vi "myRIO_BRig_RT_dataMTrig_main__NoExp.vi"(0 "input_dataMTrig":u16[](array[numeric]), 2 "input_Audio_trig_L":bool, 3 "input_Audio_trig_R":bool, 4 "input_Laser_trig":bool, 5 "input_CueLed":bool) -> (14 "output_dataMTrig":u16[](array[numeric]), 16 "output_Audio_L":bool, 17 "output_Audio_R":bool, 18 "output_Laser":bool, 19 "output_CueLed":bool)   [LabVIEW 2014]
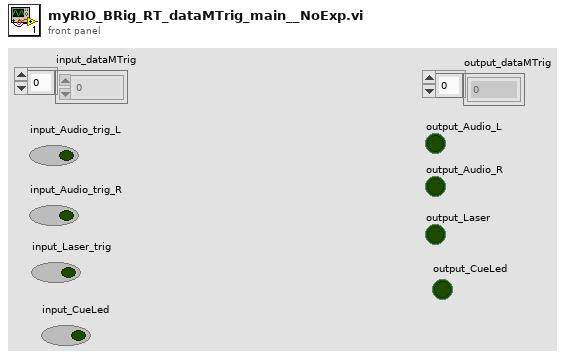
[diagram p1: front panel]
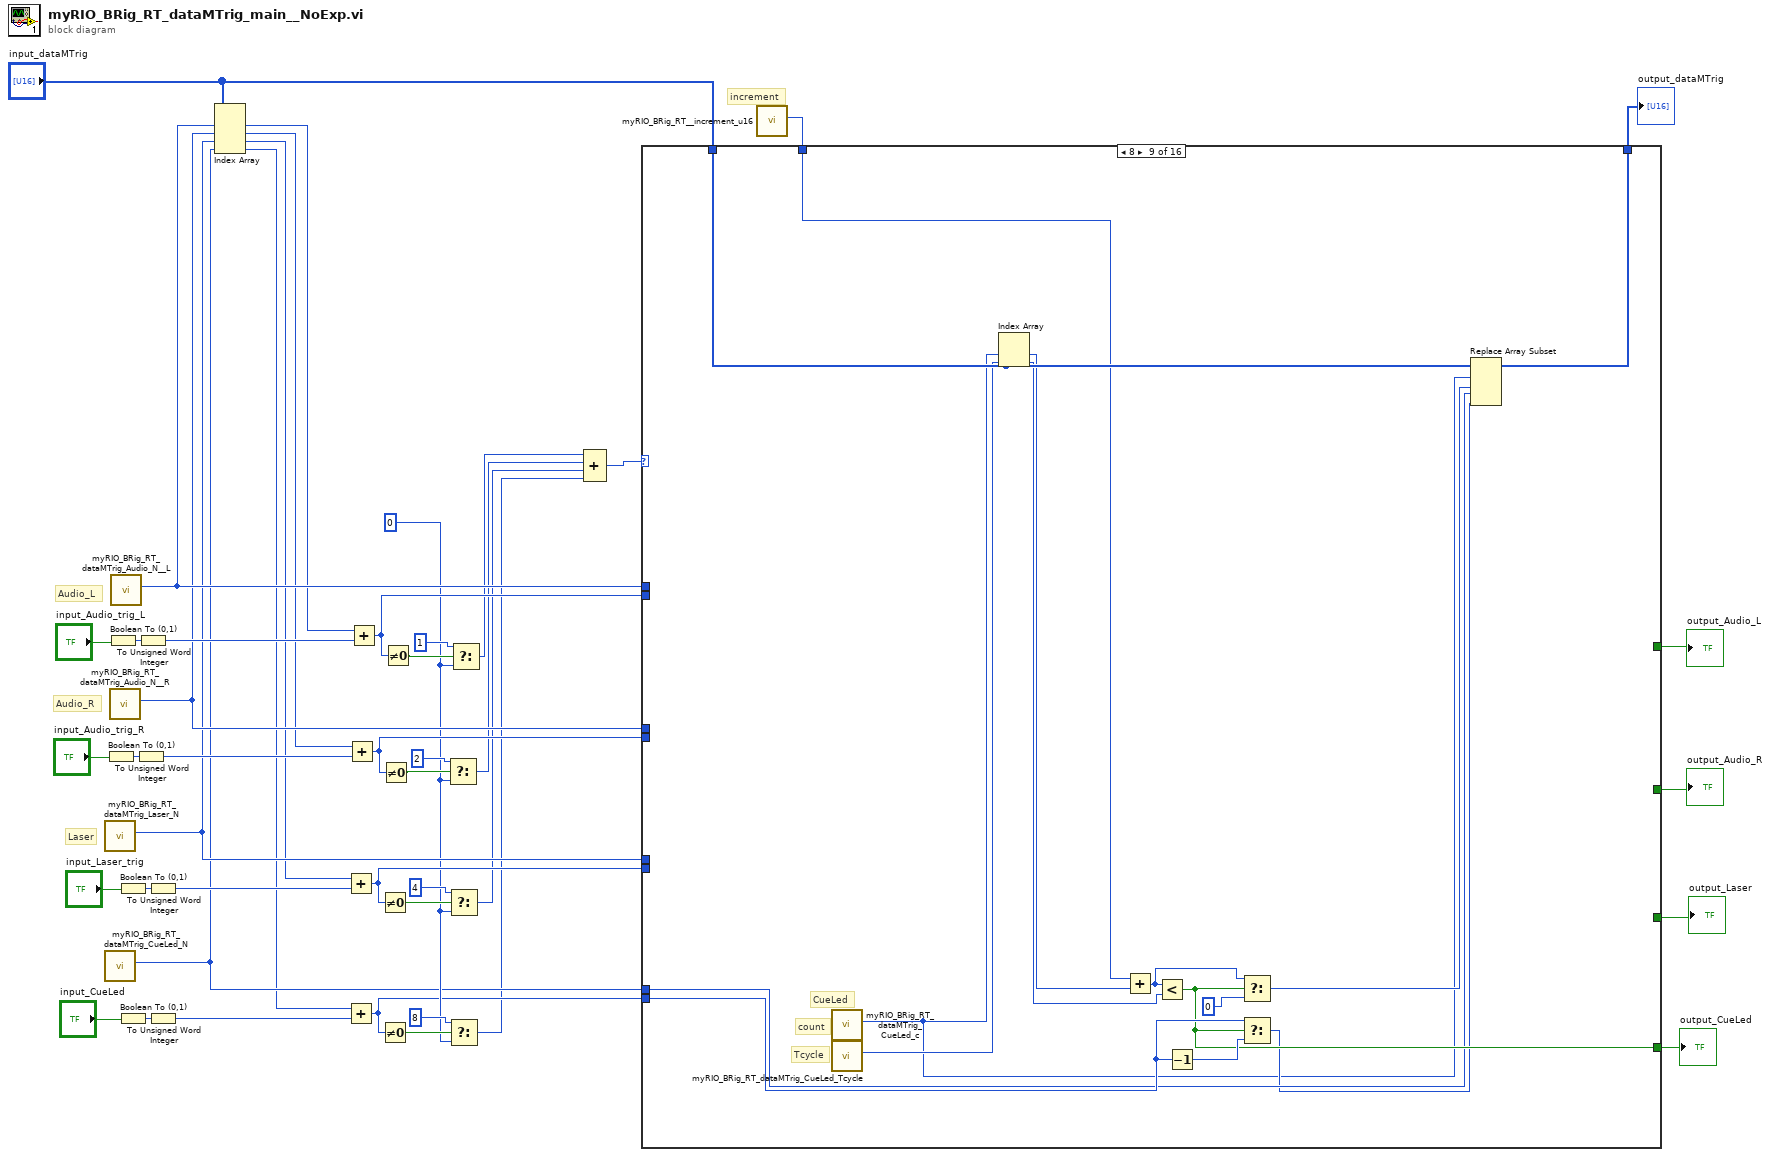
[diagram p0: block diagram]
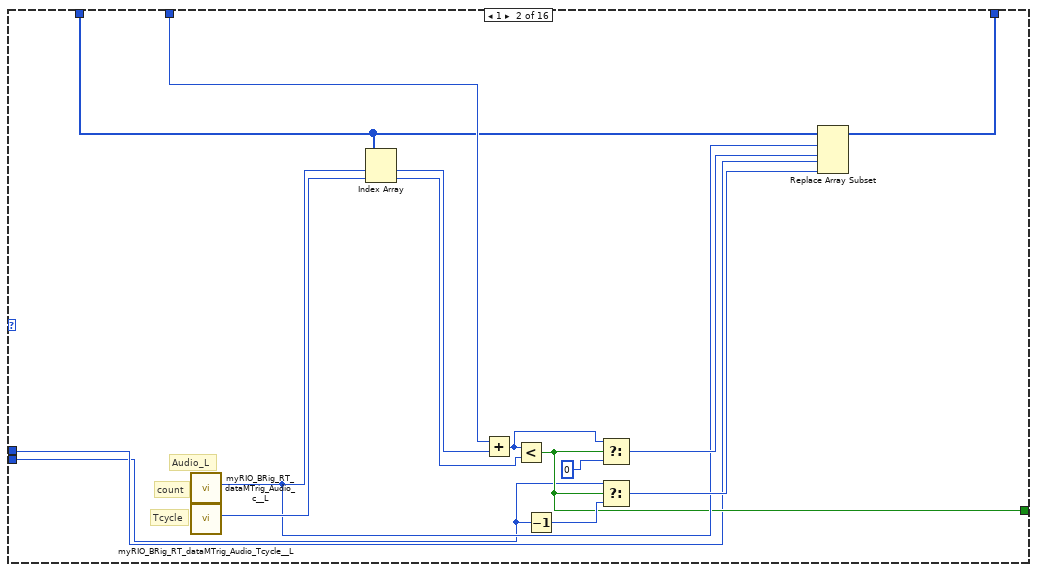
[diagram p3: hidden frame]
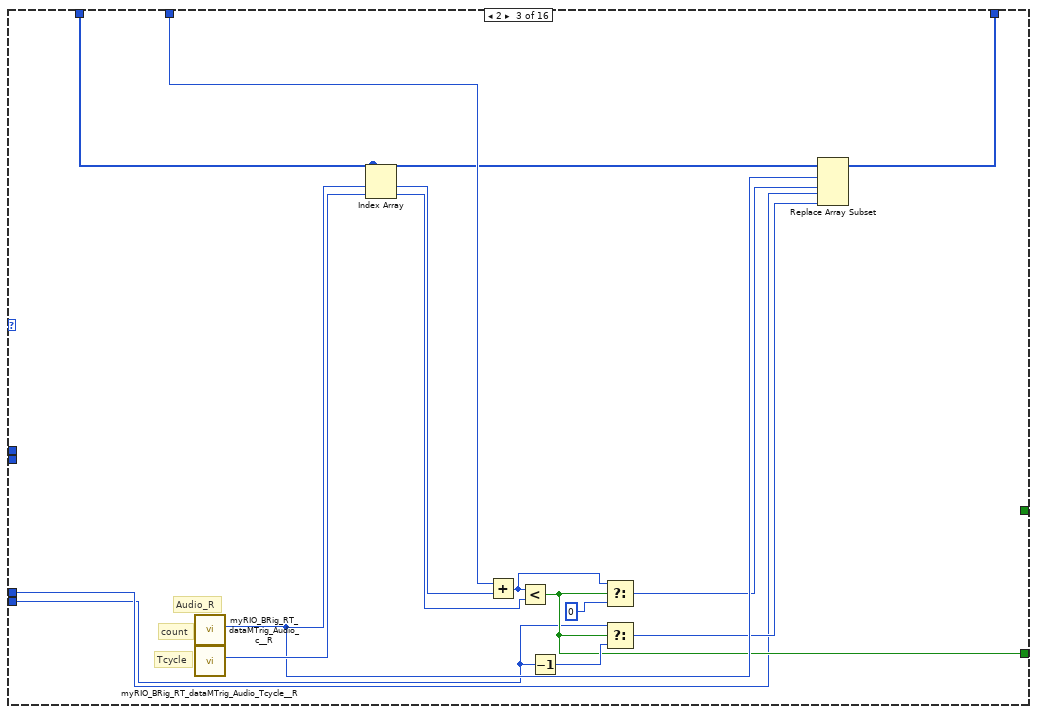
[diagram p4: hidden frame]
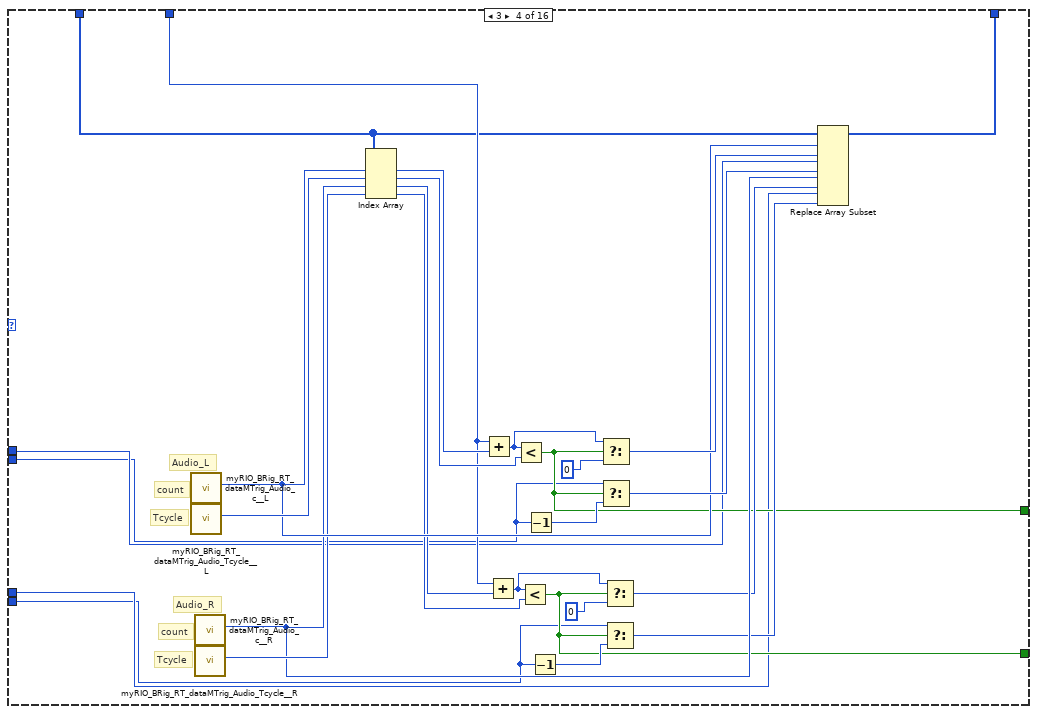
[diagram p5: hidden frame]
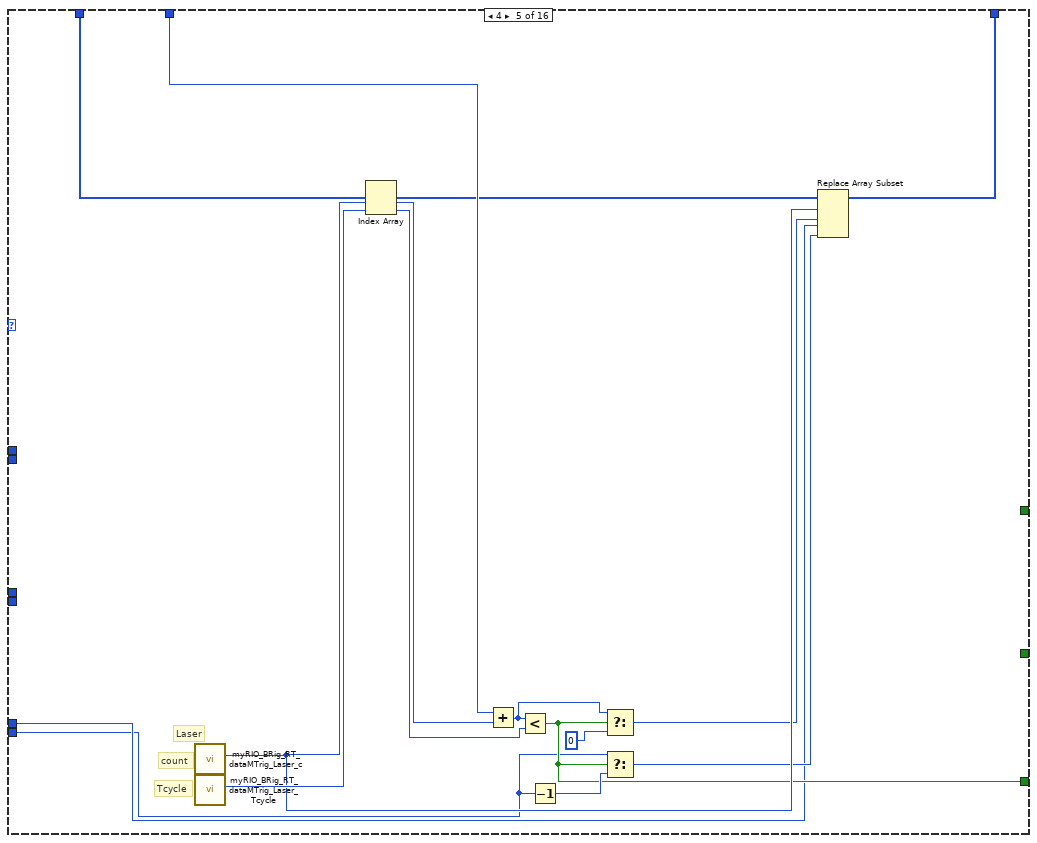
[diagram p6: hidden frame]
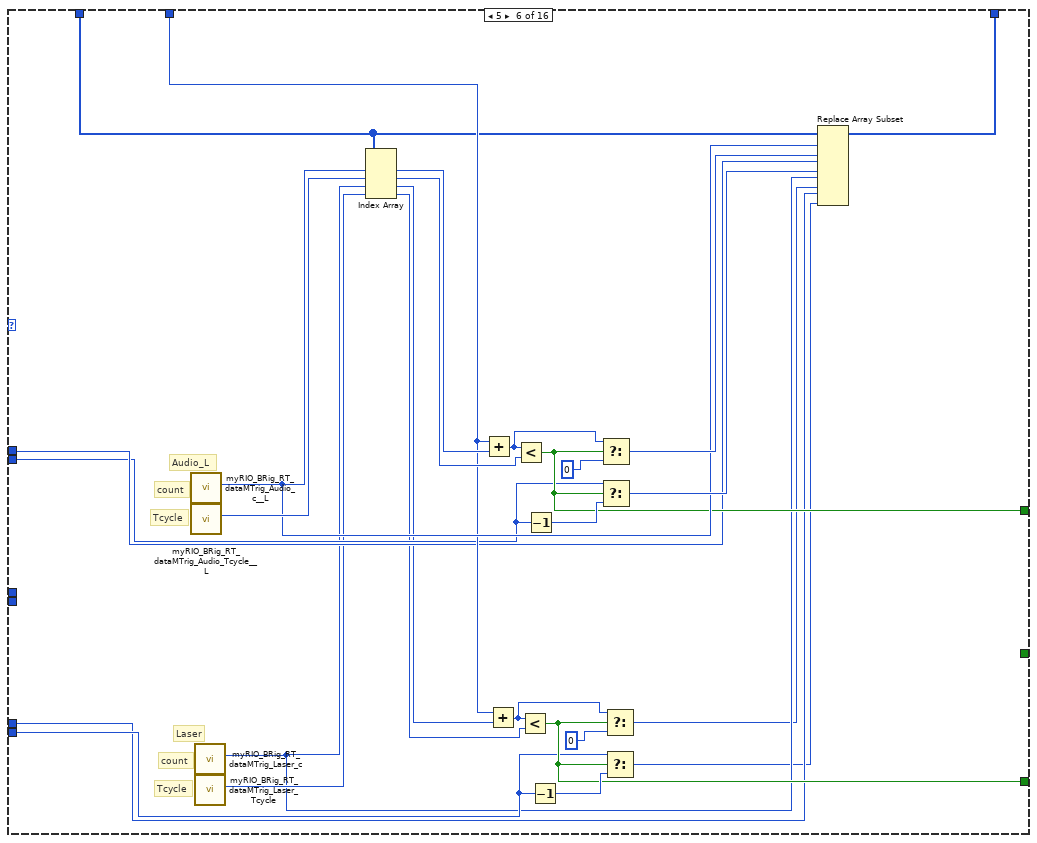
[diagram p7: hidden frame]
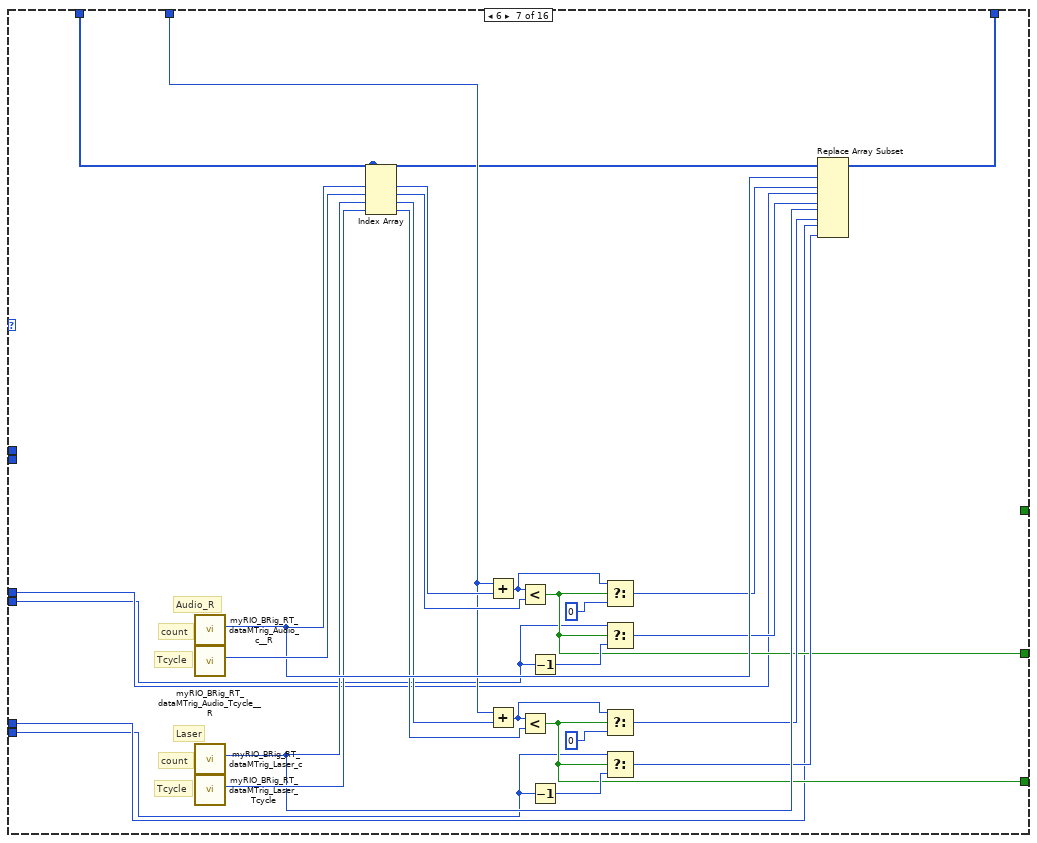
[diagram p8: hidden frame]
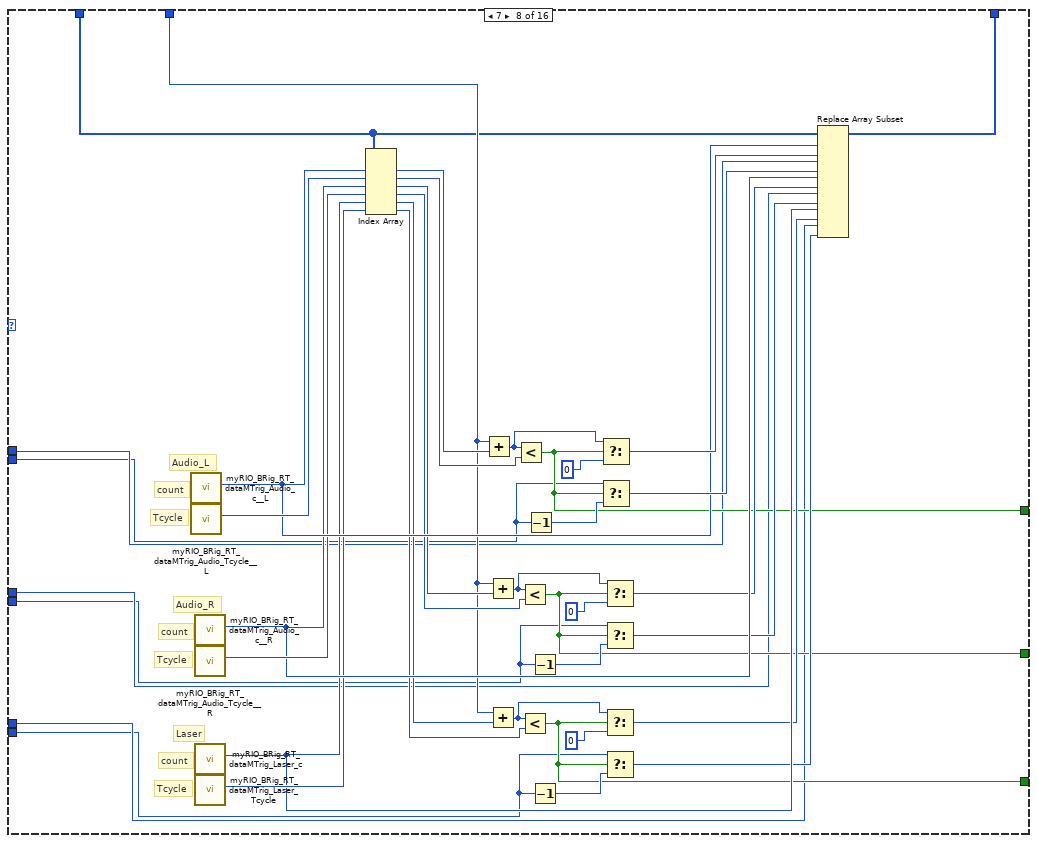
[diagram p9: hidden frame]
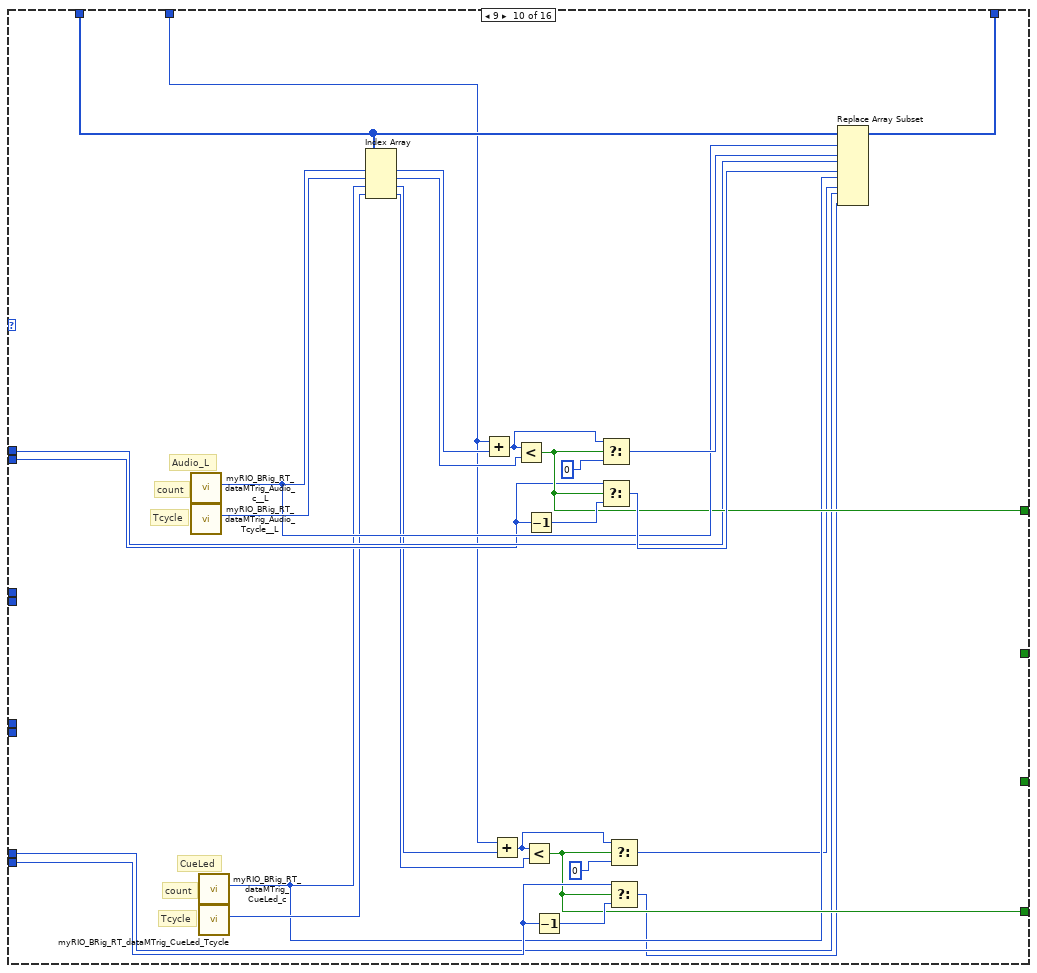
[diagram p10: hidden frame]
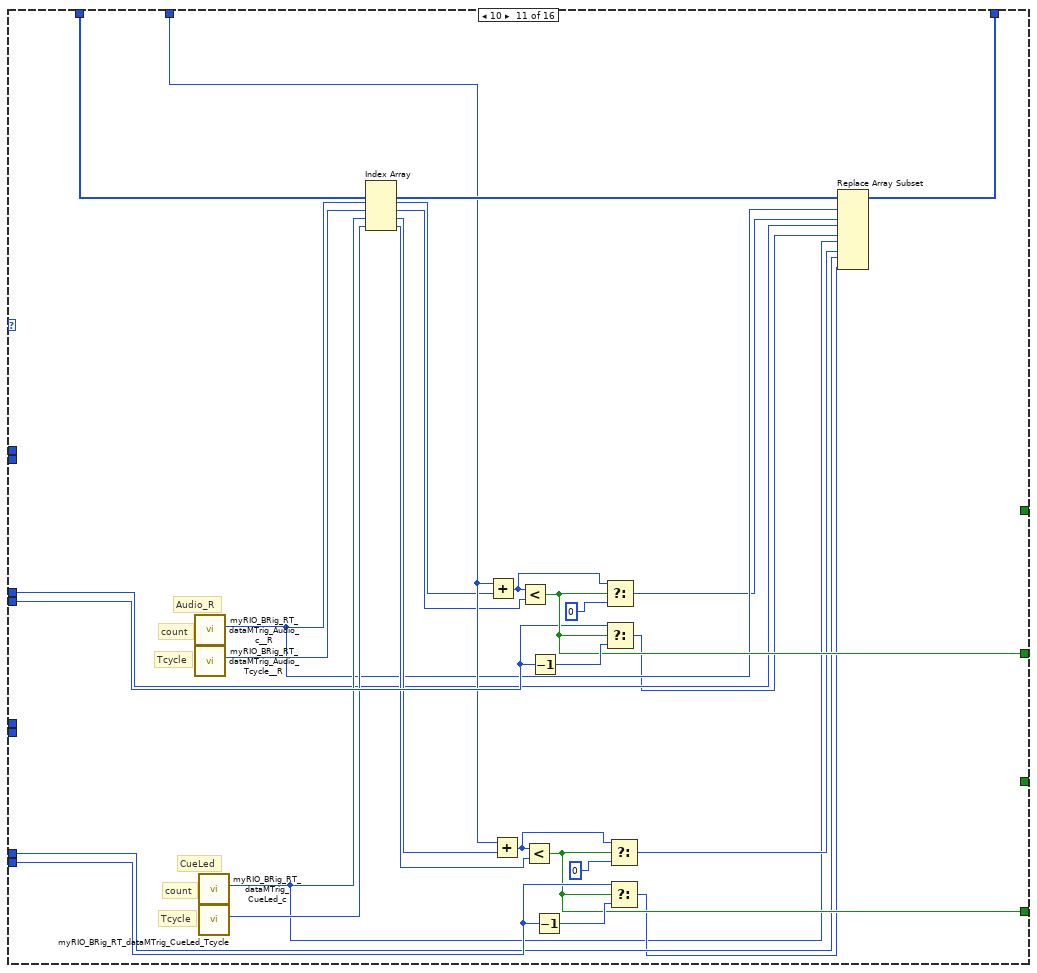
[diagram p11: hidden frame]
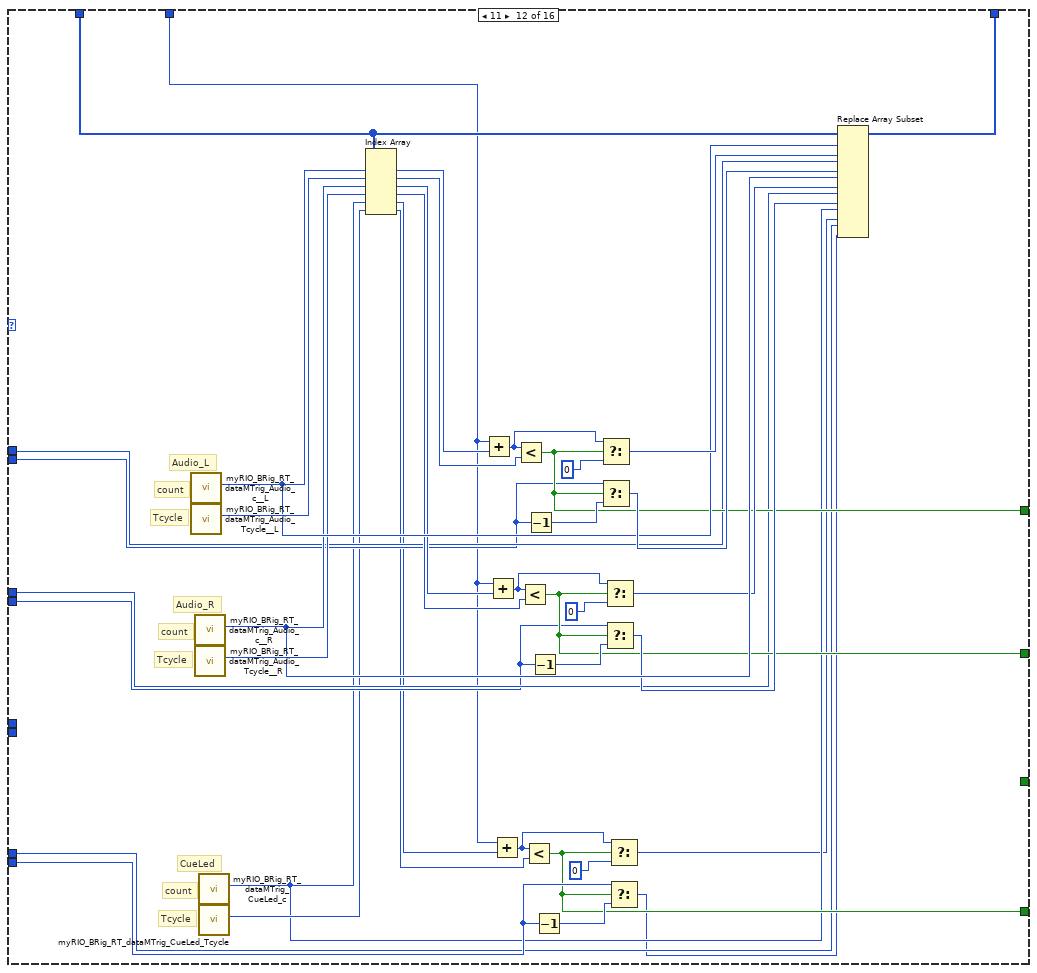
[diagram p12: hidden frame]
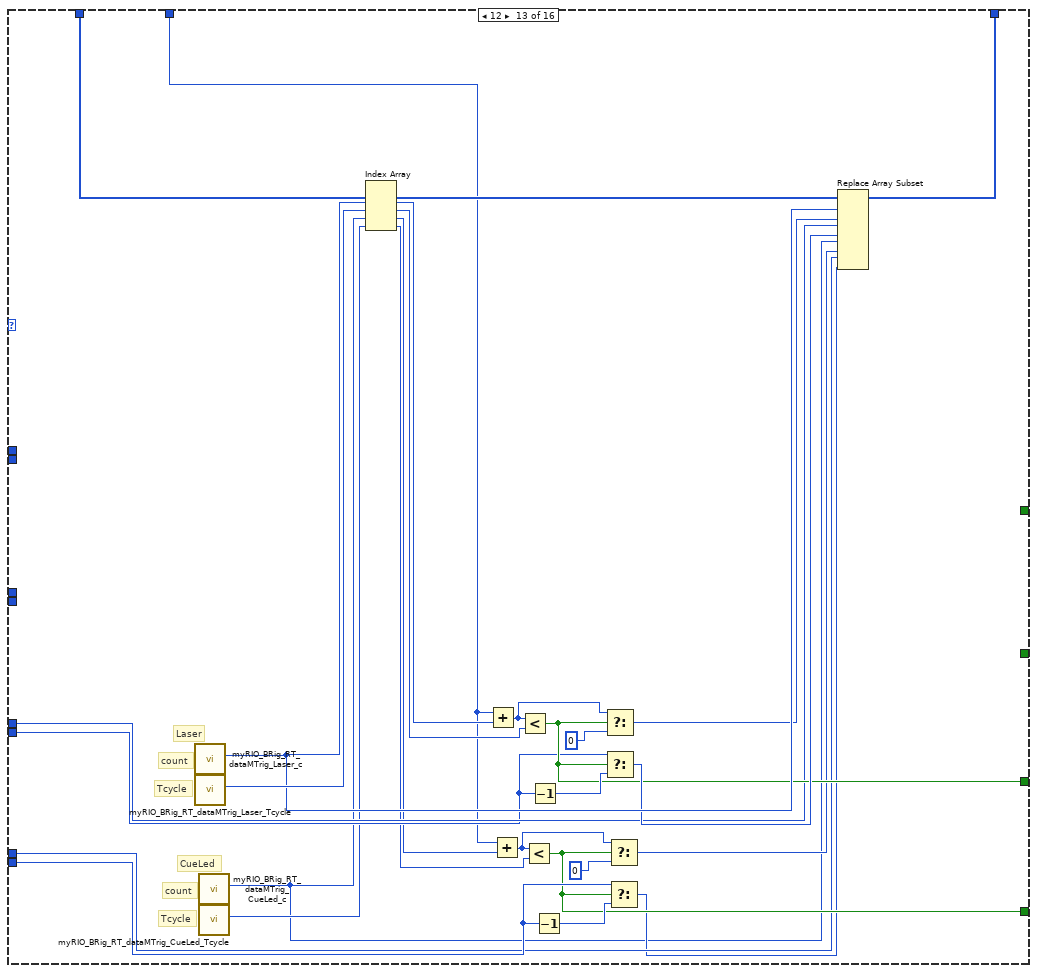
[diagram p13: hidden frame]
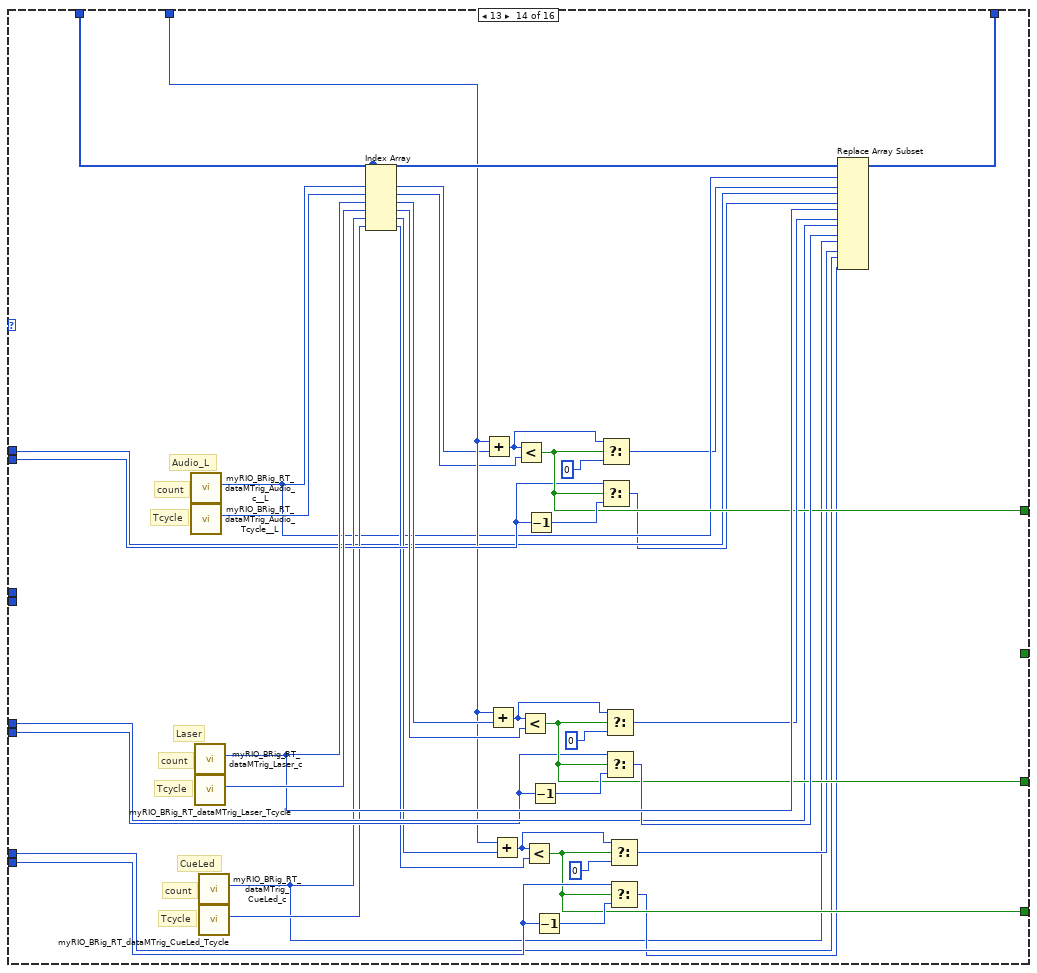
[diagram p14: hidden frame]
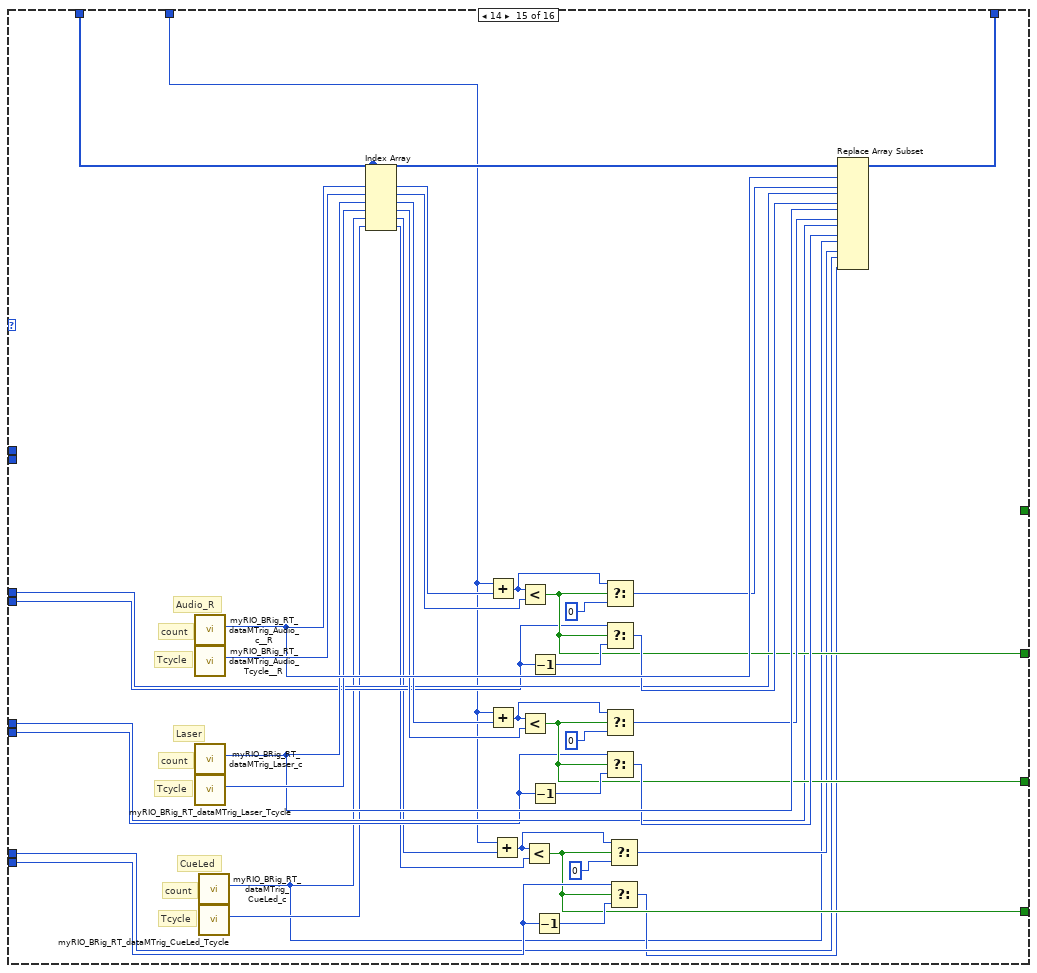
[diagram p15: hidden frame]
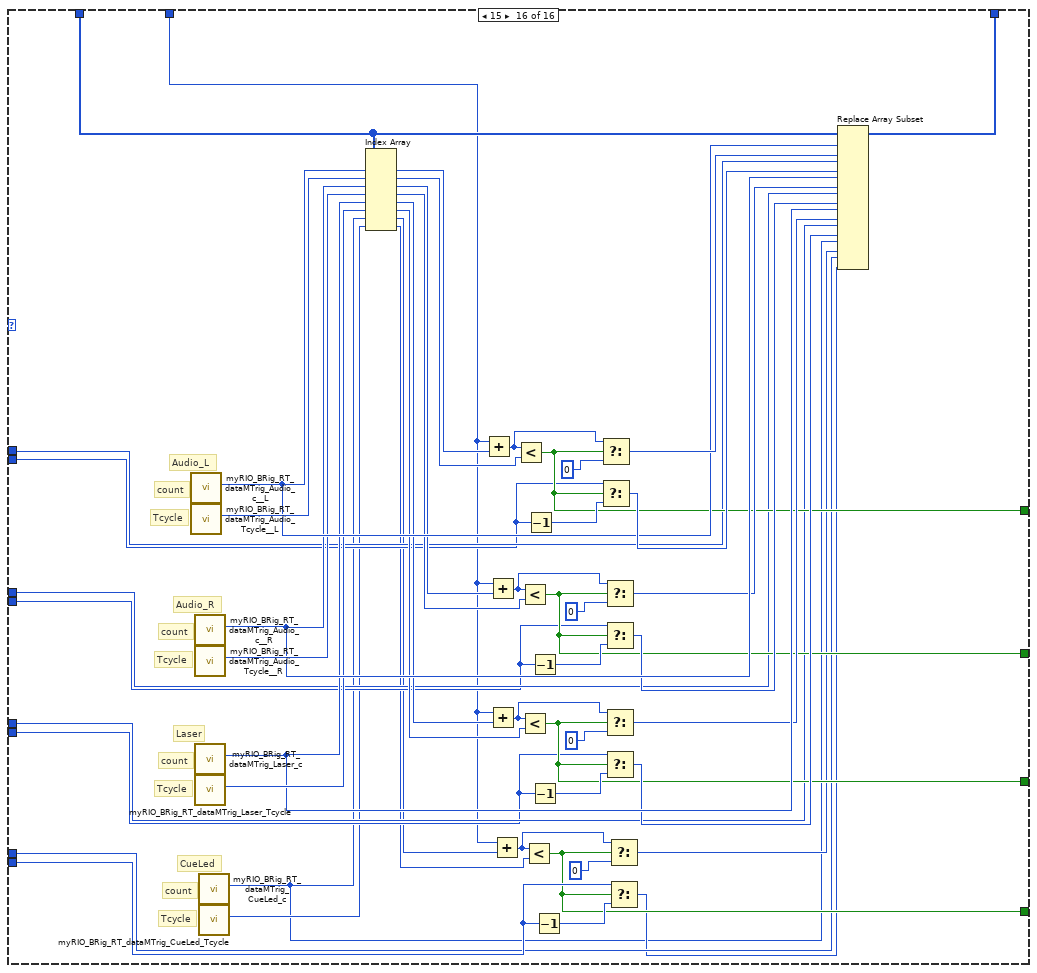
[diagram p16: hidden frame]
diagram:
  w8 = u8 0 ("f")
  # "Laser"
  # "Audio_R"
  # "increment"
  # "Audio_L"
  n1 = call "myRIO_BRig_RT_dataMTrig_Laser_N.vi"() -> ("output_Laser_N"=w17:i32)  [unwired: 11 in]
  n2 = call "myRIO_BRig_RT_dataMTrig_CueLed_N.vi"() -> ("output_CueLed_N"=w4:i32)  [unwired: 11 in]
  n3 = Boolean To (0,1)(Boolean="input_Audio_trig_R") -> (0, 1=w33:i16)
  n4 = Boolean To (0,1)(Boolean="input_Audio_trig_L") -> (0, 1=w45:i16)
  n5 = call "myRIO_BRig_RT_dataMTrig_Audio_N__R.vi"() -> ("output_Audio_N__R"=w27:i32)  [unwired: 11 in]
  n6 = call "myRIO_BRig_RT_dataMTrig_Audio_N__L.vi"() -> ("output_Audio_N__L"=w28:i32)  [unwired: 11 in]
  n7 = Boolean To (0,1)(Boolean="input_Laser_trig") -> (0, 1=w23:i16)
  n8 = Boolean To (0,1)(Boolean="input_CueLed") -> (0, 1=w12:i16)
  n9 = To Unsigned Word Integer(number=w33) -> (unsigned 16bit integer=w32:u16)
  n10 = To Unsigned Word Integer(number=w45) -> (unsigned 16bit integer=w44:u16)
  n11 = To Unsigned Word Integer(number=w23) -> (unsigned 16bit integer=w21:u16)
  n12 = To Unsigned Word Integer(number=w12) -> (unsigned 16bit integer=w11:u16)
  n13 = Index Array(array="input_dataMTrig", index #1=w28, index #2=w27, index #3=w17, index #4=w4) -> (element #1=w26:u16, element #2=w25:u16, element #3=w6:u16, element #4=w3:u16)
  n14 = Add(x=w6, y=w21) -> (x+y=w18:u16)
  n15 = Add(x=w3, y=w11) -> (x+y=w5:u16)
  n16 = Add(x=w25, y=w32) -> (x+y=w29:u16)
  n17 = Add(x=w26, y=w44) -> (x+y=w37:u16)
  n18 = Not Equal To 0?(x=w18) -> (x != 0?=w19:bool)
  n19 = Not Equal To 0?(x=w5) -> (x != 0?=w9:bool)
  n20 = Not Equal To 0?(x=w29) -> (x != 0?=w30:bool)
  n21 = Not Equal To 0?(x=w37) -> (x != 0?=w42:bool)
  n22 = Select(t=u8 2, s=w30, f=w8) -> (s? t:f=w15:u8)
  n23 = Select(t=u8 4, s=w19, f=w8) -> (s? t:f=w14:u8)
  n24 = Select(t=u8 8, s=w9, f=w8) -> (s? t:f=w2:u8)
  n25 = Select(t=u8 1, s=w42, f=w8) -> (s? t:f=w16:u8)
  n26 = Compound Arithmetic op=ADD(w16, w15, w14, w2) -> (w13:u8)
  n27 = call "myRIO_BRig_RT__increment_u16.vi"() -> ("output_increment__u16"=w40:u16)  [unwired: 11 in]
  n28 = case shown="8" w13 {
    tunnel: "input_dataMTrig" -> [w46 w51 w66 w84 w108 w132 w153 w183 w226 w244 w277 w301 w337 w373 w406 w448]
    tunnel: w40 -> [_ w52 w67 w85 w109 w133 w154 w184 w214 w234 w263 w288 w322 w356 w388 w427]
    tunnel: [w46 w50 w65 w83 w107 w131 w152 w182 w225 w243 w276 w300 w336 w372 w405 w447] -> w39
    tunnel: w28 -> [_ w48 _ w80 _ w128 _ w178 _ w241 _ w297 _ w348 _ w443]
    tunnel: w37 -> [_ w47 _ w79 _ w127 _ w177 _ w240 _ w296 _ w369 _ w442]
    tunnel: [_ w49 _ w82 _ w130 _ w181 _ w242 _ w299 _ w371 _ w446] -> w36
    tunnel: [_ _ w64 w81 _ _ w151 w180 _ _ w275 w298 _ _ w404 w445] -> w35
    tunnel: [_ _ _ _ w106 w129 w150 w179 _ _ _ _ w335 w370 w403 w444] -> w34
    tunnel: w27 -> [_ _ w63 w78 _ _ w149 w176 _ _ w255 w295 _ _ w402 w441]
    tunnel: w29 -> [_ _ w62 w77 _ _ w148 w175 _ _ w274 w294 _ _ w401 w440]
    tunnel: w17 -> [_ _ _ _ w105 w120 w147 w174 _ _ _ _ w334 w368 w400 w439]
    tunnel: w18 -> [_ _ _ _ w104 w126 w146 w173 _ _ _ _ w333 w367 w399 w438]
    tunnel: w4 -> [_ _ _ _ _ _ _ _ w219 w228 w268 w282 w327 w361 w393 w432]
    tunnel: w5 -> [_ _ _ _ _ _ _ _ w221 w236 w270 w290 w329 w363 w395 w434]
    tunnel: [_ _ _ _ _ _ _ _ w220 w235 w269 w289 w328 w362 w394 w433] -> w1
    frame 0, Default {
    }
    frame 1 {
      # "Audio_L"
      # "Tcycle"
      # "count"
      n29 = call "myRIO_BRig_RT_dataMTrig_Audio_c__L.vi"() -> ("output_Audio_c__L"=w53:i32)  [unwired: 11 in]
      n30 = call "myRIO_BRig_RT_dataMTrig_Audio_Tcycle__L.vi"() -> ("output_Audio_Tcycle__L"=w58:i32)  [unwired: 11 in]
      n31 = Index Array(array=w51, index #1=w53, index #2=w58) -> (element #1=w57:u16, element #2=w56:u16)
      n32 = Add(x=w52, y=w57) -> (x+y=w60:u16)
      n33 = Less?(x=w60, y=w56) -> (x < y?=w49:bool)
      n34 = Decrement(x=w47) -> (x-1=w61:u16)
      n35 = Select(t=w60, s=w49, f=u16 0) -> (s? t:f=w55:u16)
      n36 = Select(t=w47, s=w49, f=w61) -> (s? t:f=w54:u16)
      n37 = Replace Array Subset(array=w51, new element #1=w55, index #1=w53, new element #2=w54, index #2=w48) -> (w50:u16[])
    }
    frame 2 {
      # "Audio_R"
      # "Tcycle"
      # "count"
      n38 = call "myRIO_BRig_RT_dataMTrig_Audio_c__R.vi"() -> ("output_Audio_c__R"=w70:i32)  [unwired: 11 in]
      n39 = call "myRIO_BRig_RT_dataMTrig_Audio_Tcycle__R.vi"() -> ("output_Audio_Tcycle__R"=w71:i32)  [unwired: 11 in]
      n40 = Index Array(array=w66, index #1=w70, index #2=w71) -> (element #1=w73:u16, element #2=w72:u16)
      n41 = Add(x=w67, y=w73) -> (x+y=w75:u16)
      n42 = Less?(x=w75, y=w72) -> (x < y?=w64:bool)
      n43 = Decrement(x=w62) -> (x-1=w76:u16)
      n44 = Select(t=w75, s=w64, f=u16 0) -> (s? t:f=w69:u16)
      n45 = Select(t=w62, s=w64, f=w76) -> (s? t:f=w68:u16)
      n46 = Replace Array Subset(array=w66, new element #1=w69, index #1=w70, new element #2=w68, index #2=w63) -> (w65:u16[])
    }
    frame 3 {
      # "Audio_R"
      # "Tcycle"
      # "count"
      # "Audio_L"
      # "Tcycle"
      # "count"
      n47 = call "myRIO_BRig_RT_dataMTrig_Audio_c__L.vi"() -> ("output_Audio_c__L"=w95:i32)  [unwired: 11 in]
      n48 = call "myRIO_BRig_RT_dataMTrig_Audio_Tcycle__L.vi"() -> ("output_Audio_Tcycle__L"=w100:i32)  [unwired: 11 in]
      n49 = call "myRIO_BRig_RT_dataMTrig_Audio_c__R.vi"() -> ("output_Audio_c__R"=w88:i32)  [unwired: 11 in]
      n50 = call "myRIO_BRig_RT_dataMTrig_Audio_Tcycle__R.vi"() -> ("output_Audio_Tcycle__R"=w89:i32)  [unwired: 11 in]
      n51 = Index Array(array=w84, index #1=w95, index #2=w100, index #3=w88, index #4=w89) -> (element #1=w99:u16, element #2=w98:u16, element #3=w91:u16, element #4=w90:u16)
      n52 = Add(x=w85, y=w99) -> (x+y=w102:u16)
      n53 = Add(x=w85, y=w91) -> (x+y=w93:u16)
      n54 = Less?(x=w102, y=w98) -> (x < y?=w82:bool)
      n55 = Less?(x=w93, y=w90) -> (x < y?=w81:bool)
      n56 = Decrement(x=w79) -> (x-1=w103:u16)
      n57 = Decrement(x=w77) -> (x-1=w94:u16)
      n58 = Select(t=w102, s=w82, f=u16 0) -> (s? t:f=w97:u16)
      n59 = Select(t=w79, s=w82, f=w103) -> (s? t:f=w96:u16)
      n60 = Select(t=w93, s=w81, f=u16 0) -> (s? t:f=w87:u16)
      n61 = Select(t=w77, s=w81, f=w94) -> (s? t:f=w86:u16)
      n62 = Replace Array Subset(array=w84, new element #1=w97, index #1=w95, new element #2=w96, index #2=w80, new element #3=w87, index #3=w88, new element #4=w86, index #4=w78) -> (w83:u16[])
    }
    frame 4 {
      # "Laser"
      # "Tcycle"
      # "count"
      n63 = call "myRIO_BRig_RT_dataMTrig_Laser_c.vi"() -> ("output_Laser_c"=w112:i32)  [unwired: 11 in]
      n64 = call "myRIO_BRig_RT_dataMTrig_Laser_Tcycle.vi"() -> ("output_Laser_Tcycle"=w115:i32)  [unwired: 11 in]
      n65 = Index Array(array=w108, index #1=w112, index #2=w115) -> (element #1=w114:u16, element #2=w113:u16)
      n66 = Add(x=w109, y=w114) -> (x+y=w117:u16)
      n67 = Less?(x=w117, y=w113) -> (x < y?=w106:bool)
      n68 = Decrement(x=w104) -> (x-1=w118:u16)
      n69 = Select(t=w117, s=w106, f=u16 0) -> (s? t:f=w111:u16)
      n70 = Select(t=w104, s=w106, f=w118) -> (s? t:f=w110:u16)
      n71 = Replace Array Subset(array=w108, new element #1=w111, index #1=w112, new element #2=w110, index #2=w105) -> (w107:u16[])
    }
    frame 5 {
      # "Laser"
      # "Tcycle"
      # "count"
      # "Audio_L"
      # "Tcycle"
      # "count"
      n72 = call "myRIO_BRig_RT_dataMTrig_Audio_c__L.vi"() -> ("output_Audio_c__L"=w137:i32)  [unwired: 11 in]
      n73 = call "myRIO_BRig_RT_dataMTrig_Audio_Tcycle__L.vi"() -> ("output_Audio_Tcycle__L"=w142:i32)  [unwired: 11 in]
      n74 = call "myRIO_BRig_RT_dataMTrig_Laser_c.vi"() -> ("output_Laser_c"=w122:i32)  [unwired: 11 in]
      n75 = call "myRIO_BRig_RT_dataMTrig_Laser_Tcycle.vi"() -> ("output_Laser_Tcycle"=w125:i32)  [unwired: 11 in]
      n76 = Index Array(array=w132, index #1=w137, index #2=w142, index #3=w122, index #4=w125) -> (element #1=w141:u16, element #2=w140:u16, element #3=w124:u16, element #4=w123:u16)
      n77 = Add(x=w133, y=w141) -> (x+y=w144:u16)
      n78 = Add(x=w133, y=w124) -> (x+y=w135:u16)
      n79 = Less?(x=w144, y=w140) -> (x < y?=w130:bool)
      n80 = Less?(x=w135, y=w123) -> (x < y?=w129:bool)
      n81 = Decrement(x=w127) -> (x-1=w145:u16)
      n82 = Decrement(x=w126) -> (x-1=w136:u16)
      n83 = Select(t=w144, s=w130, f=u16 0) -> (s? t:f=w139:u16)
      n84 = Select(t=w127, s=w130, f=w145) -> (s? t:f=w138:u16)
      n85 = Select(t=w135, s=w129, f=u16 0) -> (s? t:f=w121:u16)
      n86 = Select(t=w126, s=w129, f=w136) -> (s? t:f=w119:u16)
      n87 = Replace Array Subset(array=w132, new element #1=w139, index #1=w137, new element #2=w138, index #2=w128, new element #3=w121, index #3=w122, new element #4=w119, index #4=w120) -> (w131:u16[])
    }
    frame 6 {
      # "Laser"
      # "Tcycle"
      # "count"
      # "Audio_R"
      # "Tcycle"
      # "count"
      n88 = call "myRIO_BRig_RT_dataMTrig_Audio_c__R.vi"() -> ("output_Audio_c__R"=w166:i32)  [unwired: 11 in]
      n89 = call "myRIO_BRig_RT_dataMTrig_Audio_Tcycle__R.vi"() -> ("output_Audio_Tcycle__R"=w167:i32)  [unwired: 11 in]
      n90 = call "myRIO_BRig_RT_dataMTrig_Laser_c.vi"() -> ("output_Laser_c"=w157:i32)  [unwired: 11 in]
      n91 = call "myRIO_BRig_RT_dataMTrig_Laser_Tcycle.vi"() -> ("output_Laser_Tcycle"=w160:i32)  [unwired: 11 in]
      n92 = Index Array(array=w153, index #1=w166, index #2=w167, index #3=w157, index #4=w160) -> (element #1=w169:u16, element #2=w168:u16, element #3=w159:u16, element #4=w158:u16)
      n93 = Add(x=w154, y=w169) -> (x+y=w171:u16)
      n94 = Add(x=w154, y=w159) -> (x+y=w162:u16)
      n95 = Less?(x=w171, y=w168) -> (x < y?=w151:bool)
      n96 = Less?(x=w162, y=w158) -> (x < y?=w150:bool)
      n97 = Decrement(x=w148) -> (x-1=w172:u16)
      n98 = Decrement(x=w146) -> (x-1=w163:u16)
      n99 = Select(t=w171, s=w151, f=u16 0) -> (s? t:f=w165:u16)
      n100 = Select(t=w148, s=w151, f=w172) -> (s? t:f=w164:u16)
      n101 = Select(t=w162, s=w150, f=u16 0) -> (s? t:f=w156:u16)
      n102 = Select(t=w146, s=w150, f=w163) -> (s? t:f=w155:u16)
      n103 = Replace Array Subset(array=w153, new element #1=w165, index #1=w166, new element #2=w164, index #2=w149, new element #3=w156, index #3=w157, new element #4=w155, index #4=w147) -> (w152:u16[])
    }
    frame 7 {
      # "Laser"
      # "Tcycle"
      # "count"
      # "Audio_R"
      # "Tcycle"
      # "count"
      # "Audio_L"
      # "Tcycle"
      # "count"
      n104 = call "myRIO_BRig_RT_dataMTrig_Audio_c__L.vi"() -> ("output_Audio_c__L"=w203:i32)  [unwired: 11 in]
      n105 = call "myRIO_BRig_RT_dataMTrig_Audio_Tcycle__L.vi"() -> ("output_Audio_Tcycle__L"=w208:i32)  [unwired: 11 in]
      n106 = call "myRIO_BRig_RT_dataMTrig_Audio_c__R.vi"() -> ("output_Audio_c__R"=w196:i32)  [unwired: 11 in]
      n107 = call "myRIO_BRig_RT_dataMTrig_Audio_Tcycle__R.vi"() -> ("output_Audio_Tcycle__R"=w197:i32)  [unwired: 11 in]
      n108 = call "myRIO_BRig_RT_dataMTrig_Laser_c.vi"() -> ("output_Laser_c"=w187:i32)  [unwired: 11 in]
      n109 = call "myRIO_BRig_RT_dataMTrig_Laser_Tcycle.vi"() -> ("output_Laser_Tcycle"=w190:i32)  [unwired: 11 in]
      n110 = Index Array(array=w183, index #1=w203, index #2=w208, index #3=w196, index #4=w197, index #5=w187, index #6=w190) -> (element #1=w207:u16, element #2=w206:u16, element #3=w199:u16, element #4=w198:u16, element #5=w189:u16, element #6=w188:u16)
      n111 = Add(x=w184, y=w207) -> (x+y=w210:u16)
      n112 = Add(x=w184, y=w199) -> (x+y=w201:u16)
      n113 = Add(x=w184, y=w189) -> (x+y=w192:u16)
      n114 = Less?(x=w210, y=w206) -> (x < y?=w181:bool)
      n115 = Less?(x=w201, y=w198) -> (x < y?=w180:bool)
      n116 = Less?(x=w192, y=w188) -> (x < y?=w179:bool)
      n117 = Decrement(x=w177) -> (x-1=w211:u16)
      n118 = Decrement(x=w175) -> (x-1=w202:u16)
      n119 = Decrement(x=w173) -> (x-1=w193:u16)
      n120 = Select(t=w210, s=w181, f=u16 0) -> (s? t:f=w205:u16)
      n121 = Select(t=w177, s=w181, f=w211) -> (s? t:f=w204:u16)
      n122 = Select(t=w201, s=w180, f=u16 0) -> (s? t:f=w195:u16)
      n123 = Select(t=w175, s=w180, f=w202) -> (s? t:f=w194:u16)
      n124 = Select(t=w192, s=w179, f=u16 0) -> (s? t:f=w186:u16)
      n125 = Select(t=w173, s=w179, f=w193) -> (s? t:f=w185:u16)
      n126 = Replace Array Subset(array=w183, new element #1=w205, index #1=w203, new element #2=w204, index #2=w178, new element #3=w195, index #3=w196, new element #4=w194, index #4=w176, new element #5=w186, index #5=w187, new element #6=w185, index #6=w174) -> (w182:u16[])
    }
    frame 8 {
      # "CueLed"
      # "Tcycle"
      # "count"
      n127 = call "myRIO_BRig_RT_dataMTrig_CueLed_c.vi"() -> ("output_CueLed_c"=w212:i32)  [unwired: 11 in]
      n128 = call "myRIO_BRig_RT_dataMTrig_CueLed_Tcycle.vi"() -> ("output_CueLed_Tcycle"=w213:i32)  [unwired: 11 in]
      n129 = Index Array(array=w226, index #1=w212, index #2=w213) -> (element #1=w216:u16, element #2=w215:u16)
      n130 = Add(x=w214, y=w216) -> (x+y=w223:u16)
      n131 = Less?(x=w223, y=w215) -> (x < y?=w220:bool)
      n132 = Decrement(x=w221) -> (x-1=w224:u16)
      n133 = Select(t=w223, s=w220, f=u16 0) -> (s? t:f=w218:u16)
      n134 = Select(t=w221, s=w220, f=w224) -> (s? t:f=w217:u16)
      n135 = Replace Array Subset(array=w226, new element #1=w218, index #1=w212, new element #2=w217, index #2=w219) -> (w225:u16[])
    }
    frame 9 {
      # "CueLed"
      # "Tcycle"
      # "count"
      # "Audio_L"
      # "Tcycle"
      # "count"
      n136 = call "myRIO_BRig_RT_dataMTrig_Audio_c__L.vi"() -> ("output_Audio_c__L"=w245:i32)  [unwired: 11 in]
      n137 = call "myRIO_BRig_RT_dataMTrig_Audio_Tcycle__L.vi"() -> ("output_Audio_Tcycle__L"=w250:i32)  [unwired: 11 in]
      n138 = call "myRIO_BRig_RT_dataMTrig_CueLed_c.vi"() -> ("output_CueLed_c"=w230:i32)  [unwired: 11 in]
      n139 = call "myRIO_BRig_RT_dataMTrig_CueLed_Tcycle.vi"() -> ("output_CueLed_Tcycle"=w233:i32)  [unwired: 11 in]
      n140 = Index Array(array=w244, index #1=w245, index #2=w250, index #3=w230, index #4=w233) -> (element #1=w249:u16, element #2=w248:u16, element #3=w232:u16, element #4=w231:u16)
      n141 = Add(x=w234, y=w249) -> (x+y=w252:u16)
      n142 = Add(x=w234, y=w232) -> (x+y=w238:u16)
      n143 = Less?(x=w252, y=w248) -> (x < y?=w242:bool)
      n144 = Less?(x=w238, y=w231) -> (x < y?=w235:bool)
      n145 = Decrement(x=w240) -> (x-1=w253:u16)
      n146 = Decrement(x=w236) -> (x-1=w239:u16)
      n147 = Select(t=w252, s=w242, f=u16 0) -> (s? t:f=w247:u16)
      n148 = Select(t=w240, s=w242, f=w253) -> (s? t:f=w246:u16)
      n149 = Select(t=w238, s=w235, f=u16 0) -> (s? t:f=w229:u16)
      n150 = Select(t=w236, s=w235, f=w239) -> (s? t:f=w227:u16)
      n151 = Replace Array Subset(array=w244, new element #1=w247, index #1=w245, new element #2=w246, index #2=w241, new element #3=w229, index #3=w230, new element #4=w227, index #4=w228) -> (w243:u16[])
    }
    frame 10 {
      # "CueLed"
      # "Tcycle"
      # "count"
      # "Audio_R"
      # "Tcycle"
      # "count"
      n152 = call "myRIO_BRig_RT_dataMTrig_Audio_c__R.vi"() -> ("output_Audio_c__R"=w257:i32)  [unwired: 11 in]
      n153 = call "myRIO_BRig_RT_dataMTrig_Audio_Tcycle__R.vi"() -> ("output_Audio_Tcycle__R"=w260:i32)  [unwired: 11 in]
      n154 = call "myRIO_BRig_RT_dataMTrig_CueLed_c.vi"() -> ("output_CueLed_c"=w261:i32)  [unwired: 11 in]
      n155 = call "myRIO_BRig_RT_dataMTrig_CueLed_Tcycle.vi"() -> ("output_CueLed_Tcycle"=w262:i32)  [unwired: 11 in]
      n156 = Index Array(array=w277, index #1=w257, index #2=w260, index #3=w261, index #4=w262) -> (element #1=w259:u16, element #2=w258:u16, element #3=w265:u16, element #4=w264:u16)
      n157 = Add(x=w263, y=w259) -> (x+y=w279:u16)
      n158 = Add(x=w263, y=w265) -> (x+y=w272:u16)
      n159 = Less?(x=w279, y=w258) -> (x < y?=w275:bool)
      n160 = Less?(x=w272, y=w264) -> (x < y?=w269:bool)
      n161 = Decrement(x=w274) -> (x-1=w280:u16)
      n162 = Decrement(x=w270) -> (x-1=w273:u16)
      n163 = Select(t=w279, s=w275, f=u16 0) -> (s? t:f=w256:u16)
      n164 = Select(t=w274, s=w275, f=w280) -> (s? t:f=w254:u16)
      n165 = Select(t=w272, s=w269, f=u16 0) -> (s? t:f=w267:u16)
      n166 = Select(t=w270, s=w269, f=w273) -> (s? t:f=w266:u16)
      n167 = Replace Array Subset(array=w277, new element #1=w256, index #1=w257, new element #2=w254, index #2=w255, new element #3=w267, index #3=w261, new element #4=w266, index #4=w268) -> (w276:u16[])
    }
    frame 11 {
      # "CueLed"
      # "Tcycle"
      # "count"
      # "Audio_R"
      # "Tcycle"
      # "count"
      # "Audio_L"
      # "Tcycle"
      # "count"
      n168 = call "myRIO_BRig_RT_dataMTrig_Audio_c__L.vi"() -> ("output_Audio_c__L"=w311:i32)  [unwired: 11 in]
      n169 = call "myRIO_BRig_RT_dataMTrig_Audio_Tcycle__L.vi"() -> ("output_Audio_Tcycle__L"=w316:i32)  [unwired: 11 in]
      n170 = call "myRIO_BRig_RT_dataMTrig_Audio_c__R.vi"() -> ("output_Audio_c__R"=w304:i32)  [unwired: 11 in]
      n171 = call "myRIO_BRig_RT_dataMTrig_Audio_Tcycle__R.vi"() -> ("output_Audio_Tcycle__R"=w305:i32)  [unwired: 11 in]
      n172 = call "myRIO_BRig_RT_dataMTrig_CueLed_c.vi"() -> ("output_CueLed_c"=w284:i32)  [unwired: 11 in]
      n173 = call "myRIO_BRig_RT_dataMTrig_CueLed_Tcycle.vi"() -> ("output_CueLed_Tcycle"=w287:i32)  [unwired: 11 in]
      n174 = Index Array(array=w301, index #1=w311, index #2=w316, index #3=w304, index #4=w305, index #5=w284, index #6=w287) -> (element #1=w315:u16, element #2=w314:u16, element #3=w307:u16, element #4=w306:u16, element #5=w286:u16, element #6=w285:u16)
      n175 = Add(x=w288, y=w315) -> (x+y=w318:u16)
      n176 = Add(x=w288, y=w307) -> (x+y=w309:u16)
      n177 = Add(x=w288, y=w286) -> (x+y=w292:u16)
      n178 = Less?(x=w318, y=w314) -> (x < y?=w299:bool)
      n179 = Less?(x=w309, y=w306) -> (x < y?=w298:bool)
      n180 = Less?(x=w292, y=w285) -> (x < y?=w289:bool)
      n181 = Decrement(x=w296) -> (x-1=w319:u16)
      n182 = Decrement(x=w294) -> (x-1=w310:u16)
      n183 = Decrement(x=w290) -> (x-1=w293:u16)
      n184 = Select(t=w318, s=w299, f=u16 0) -> (s? t:f=w313:u16)
      n185 = Select(t=w296, s=w299, f=w319) -> (s? t:f=w312:u16)
      n186 = Select(t=w309, s=w298, f=u16 0) -> (s? t:f=w303:u16)
      n187 = Select(t=w294, s=w298, f=w310) -> (s? t:f=w302:u16)
      n188 = Select(t=w292, s=w289, f=u16 0) -> (s? t:f=w283:u16)
      n189 = Select(t=w290, s=w289, f=w293) -> (s? t:f=w281:u16)
      n190 = Replace Array Subset(array=w301, new element #1=w313, index #1=w311, new element #2=w312, index #2=w297, new element #3=w303, index #3=w304, new element #4=w302, index #4=w295, new element #5=w283, index #5=w284, new element #6=w281, index #6=w282) -> (w300:u16[])
    }
    frame 12 {
      # "CueLed"
      # "Tcycle"
      # "count"
      # "Laser"
      # "Tcycle"
      # "count"
      n191 = call "myRIO_BRig_RT_dataMTrig_Laser_c.vi"() -> ("output_Laser_c"=w340:i32)  [unwired: 11 in]
      n192 = call "myRIO_BRig_RT_dataMTrig_Laser_Tcycle.vi"() -> ("output_Laser_Tcycle"=w343:i32)  [unwired: 11 in]
      n193 = call "myRIO_BRig_RT_dataMTrig_CueLed_c.vi"() -> ("output_CueLed_c"=w320:i32)  [unwired: 11 in]
      n194 = call "myRIO_BRig_RT_dataMTrig_CueLed_Tcycle.vi"() -> ("output_CueLed_Tcycle"=w321:i32)  [unwired: 11 in]
      n195 = Index Array(array=w337, index #1=w340, index #2=w343, index #3=w320, index #4=w321) -> (element #1=w342:u16, element #2=w341:u16, element #3=w324:u16, element #4=w323:u16)
      n196 = Add(x=w322, y=w342) -> (x+y=w345:u16)
      n197 = Add(x=w322, y=w324) -> (x+y=w331:u16)
      n198 = Less?(x=w345, y=w341) -> (x < y?=w335:bool)
      n199 = Less?(x=w331, y=w323) -> (x < y?=w328:bool)
      n200 = Decrement(x=w333) -> (x-1=w346:u16)
      n201 = Decrement(x=w329) -> (x-1=w332:u16)
      n202 = Select(t=w345, s=w335, f=u16 0) -> (s? t:f=w339:u16)
      n203 = Select(t=w333, s=w335, f=w346) -> (s? t:f=w338:u16)
      n204 = Select(t=w331, s=w328, f=u16 0) -> (s? t:f=w326:u16)
      n205 = Select(t=w329, s=w328, f=w332) -> (s? t:f=w325:u16)
      n206 = Replace Array Subset(array=w337, new element #1=w339, index #1=w340, new element #2=w338, index #2=w334, new element #3=w326, index #3=w320, new element #4=w325, index #4=w327) -> (w336:u16[])
    }
    frame 13 {
      # "CueLed"
      # "Tcycle"
      # "count"
      # "Laser"
      # "Tcycle"
      # "count"
      # "Audio_L"
      # "Tcycle"
      # "count"
      n207 = call "myRIO_BRig_RT_dataMTrig_Audio_c__L.vi"() -> ("output_Audio_c__L"=w350:i32)  [unwired: 11 in]
      n208 = call "myRIO_BRig_RT_dataMTrig_Audio_Tcycle__L.vi"() -> ("output_Audio_Tcycle__L"=w353:i32)  [unwired: 11 in]
      n209 = call "myRIO_BRig_RT_dataMTrig_Laser_c.vi"() -> ("output_Laser_c"=w376:i32)  [unwired: 11 in]
      n210 = call "myRIO_BRig_RT_dataMTrig_Laser_Tcycle.vi"() -> ("output_Laser_Tcycle"=w379:i32)  [unwired: 11 in]
      n211 = call "myRIO_BRig_RT_dataMTrig_CueLed_c.vi"() -> ("output_CueLed_c"=w354:i32)  [unwired: 11 in]
      n212 = call "myRIO_BRig_RT_dataMTrig_CueLed_Tcycle.vi"() -> ("output_CueLed_Tcycle"=w355:i32)  [unwired: 11 in]
      n213 = Index Array(array=w373, index #1=w350, index #2=w353, index #3=w376, index #4=w379, index #5=w354, index #6=w355) -> (element #1=w352:u16, element #2=w351:u16, element #3=w378:u16, element #4=w377:u16, element #5=w358:u16, element #6=w357:u16)
      n214 = Add(x=w356, y=w352) -> (x+y=w384:u16)
      n215 = Add(x=w356, y=w378) -> (x+y=w381:u16)
      n216 = Add(x=w356, y=w358) -> (x+y=w365:u16)
      n217 = Less?(x=w384, y=w351) -> (x < y?=w371:bool)
      n218 = Less?(x=w381, y=w377) -> (x < y?=w370:bool)
      n219 = Less?(x=w365, y=w357) -> (x < y?=w362:bool)
      n220 = Decrement(x=w369) -> (x-1=w385:u16)
      n221 = Decrement(x=w367) -> (x-1=w382:u16)
      n222 = Decrement(x=w363) -> (x-1=w366:u16)
      n223 = Select(t=w384, s=w371, f=u16 0) -> (s? t:f=w349:u16)
      n224 = Select(t=w369, s=w371, f=w385) -> (s? t:f=w347:u16)
      n225 = Select(t=w381, s=w370, f=u16 0) -> (s? t:f=w375:u16)
      n226 = Select(t=w367, s=w370, f=w382) -> (s? t:f=w374:u16)
      n227 = Select(t=w365, s=w362, f=u16 0) -> (s? t:f=w360:u16)
      n228 = Select(t=w363, s=w362, f=w366) -> (s? t:f=w359:u16)
      n229 = Replace Array Subset(array=w373, new element #1=w349, index #1=w350, new element #2=w347, index #2=w348, new element #3=w375, index #3=w376, new element #4=w374, index #4=w368, new element #5=w360, index #5=w354, new element #6=w359, index #6=w361) -> (w372:u16[])
    }
    frame 14 {
      # "CueLed"
      # "Tcycle"
      # "count"
      # "Laser"
      # "Tcycle"
      # "count"
      # "Audio_R"
      # "Tcycle"
      # "count"
      n230 = call "myRIO_BRig_RT_dataMTrig_Audio_c__R.vi"() -> ("output_Audio_c__R"=w418:i32)  [unwired: 11 in]
      n231 = call "myRIO_BRig_RT_dataMTrig_Audio_Tcycle__R.vi"() -> ("output_Audio_Tcycle__R"=w419:i32)  [unwired: 11 in]
      n232 = call "myRIO_BRig_RT_dataMTrig_Laser_c.vi"() -> ("output_Laser_c"=w409:i32)  [unwired: 11 in]
      n233 = call "myRIO_BRig_RT_dataMTrig_Laser_Tcycle.vi"() -> ("output_Laser_Tcycle"=w412:i32)  [unwired: 11 in]
      n234 = call "myRIO_BRig_RT_dataMTrig_CueLed_c.vi"() -> ("output_CueLed_c"=w386:i32)  [unwired: 11 in]
      n235 = call "myRIO_BRig_RT_dataMTrig_CueLed_Tcycle.vi"() -> ("output_CueLed_Tcycle"=w387:i32)  [unwired: 11 in]
      n236 = Index Array(array=w406, index #1=w418, index #2=w419, index #3=w409, index #4=w412, index #5=w386, index #6=w387) -> (element #1=w421:u16, element #2=w420:u16, element #3=w411:u16, element #4=w410:u16, element #5=w390:u16, element #6=w389:u16)
      n237 = Add(x=w388, y=w421) -> (x+y=w423:u16)
      n238 = Add(x=w388, y=w411) -> (x+y=w414:u16)
      n239 = Add(x=w388, y=w390) -> (x+y=w397:u16)
      n240 = Less?(x=w423, y=w420) -> (x < y?=w404:bool)
      n241 = Less?(x=w414, y=w410) -> (x < y?=w403:bool)
      n242 = Less?(x=w397, y=w389) -> (x < y?=w394:bool)
      n243 = Decrement(x=w401) -> (x-1=w424:u16)
      n244 = Decrement(x=w399) -> (x-1=w415:u16)
      n245 = Decrement(x=w395) -> (x-1=w398:u16)
      n246 = Select(t=w423, s=w404, f=u16 0) -> (s? t:f=w417:u16)
      n247 = Select(t=w401, s=w404, f=w424) -> (s? t:f=w416:u16)
      n248 = Select(t=w414, s=w403, f=u16 0) -> (s? t:f=w408:u16)
      n249 = Select(t=w399, s=w403, f=w415) -> (s? t:f=w407:u16)
      n250 = Select(t=w397, s=w394, f=u16 0) -> (s? t:f=w392:u16)
      n251 = Select(t=w395, s=w394, f=w398) -> (s? t:f=w391:u16)
      n252 = Replace Array Subset(array=w406, new element #1=w417, index #1=w418, new element #2=w416, index #2=w402, new element #3=w408, index #3=w409, new element #4=w407, index #4=w400, new element #5=w392, index #5=w386, new element #6=w391, index #6=w393) -> (w405:u16[])
    }
    frame 15 {
      # "CueLed"
      # "Tcycle"
      # "count"
      # "Laser"
      # "Tcycle"
      # "count"
      # "Audio_R"
      # "Tcycle"
      # "count"
      # "Audio_L"
      # "Tcycle"
      # "count"
      n253 = call "myRIO_BRig_RT_dataMTrig_Audio_c__L.vi"() -> ("output_Audio_c__L"=w467:i32)  [unwired: 11 in]
      n254 = call "myRIO_BRig_RT_dataMTrig_Audio_Tcycle__L.vi"() -> ("output_Audio_Tcycle__L"=w472:i32)  [unwired: 11 in]
      n255 = call "myRIO_BRig_RT_dataMTrig_Audio_c__R.vi"() -> ("output_Audio_c__R"=w460:i32)  [unwired: 11 in]
      n256 = call "myRIO_BRig_RT_dataMTrig_Audio_Tcycle__R.vi"() -> ("output_Audio_Tcycle__R"=w461:i32)  [unwired: 11 in]
      n257 = call "myRIO_BRig_RT_dataMTrig_Laser_c.vi"() -> ("output_Laser_c"=w451:i32)  [unwired: 11 in]
      n258 = call "myRIO_BRig_RT_dataMTrig_Laser_Tcycle.vi"() -> ("output_Laser_Tcycle"=w454:i32)  [unwired: 11 in]
      n259 = call "myRIO_BRig_RT_dataMTrig_CueLed_c.vi"() -> ("output_CueLed_c"=w425:i32)  [unwired: 11 in]
      n260 = call "myRIO_BRig_RT_dataMTrig_CueLed_Tcycle.vi"() -> ("output_CueLed_Tcycle"=w426:i32)  [unwired: 11 in]
      n261 = Index Array(array=w448, index #1=w467, index #2=w472, index #3=w460, index #4=w461, index #5=w451, index #6=w454, index #7=w425, index #8=w426) -> (element #1=w471:u16, element #2=w470:u16, element #3=w463:u16, element #4=w462:u16, element #5=w453:u16, element #6=w452:u16, element #7=w429:u16, element #8=w428:u16)
      n262 = Add(x=w427, y=w471) -> (x+y=w474:u16)
      n263 = Add(x=w427, y=w463) -> (x+y=w465:u16)
      n264 = Add(x=w427, y=w453) -> (x+y=w456:u16)
      n265 = Add(x=w427, y=w429) -> (x+y=w436:u16)
      n266 = Less?(x=w474, y=w470) -> (x < y?=w446:bool)
      n267 = Less?(x=w465, y=w462) -> (x < y?=w445:bool)
      n268 = Less?(x=w456, y=w452) -> (x < y?=w444:bool)
      n269 = Less?(x=w436, y=w428) -> (x < y?=w433:bool)
      n270 = Decrement(x=w442) -> (x-1=w475:u16)
      n271 = Decrement(x=w440) -> (x-1=w466:u16)
      n272 = Decrement(x=w438) -> (x-1=w457:u16)
      n273 = Decrement(x=w434) -> (x-1=w437:u16)
      n274 = Select(t=w474, s=w446, f=u16 0) -> (s? t:f=w469:u16)
      n275 = Select(t=w442, s=w446, f=w475) -> (s? t:f=w468:u16)
      n276 = Select(t=w465, s=w445, f=u16 0) -> (s? t:f=w459:u16)
      n277 = Select(t=w440, s=w445, f=w466) -> (s? t:f=w458:u16)
      n278 = Select(t=w456, s=w444, f=u16 0) -> (s? t:f=w450:u16)
      n279 = Select(t=w438, s=w444, f=w457) -> (s? t:f=w449:u16)
      n280 = Select(t=w436, s=w433, f=u16 0) -> (s? t:f=w431:u16)
      n281 = Select(t=w434, s=w433, f=w437) -> (s? t:f=w430:u16)
      n282 = Replace Array Subset(array=w448, new element #1=w469, index #1=w467, new element #2=w468, index #2=w443, new element #3=w459, index #3=w460, new element #4=w458, index #4=w441, new element #5=w450, index #5=w451, new element #6=w449, index #6=w439, new element #7=w431, index #7=w425, new element #8=w430, index #8=w432) -> (w447:u16[])
    }
  }
  "output_dataMTrig" <- w39
  "output_Audio_L" <- w36
  "output_Audio_R" <- w35
  "output_Laser" <- w34
  "output_CueLed" <- w1
